vi "Accept.vi"(8 "Error in (no error)":errorcluster, 10 "Log in":T1 {"Priority" items=["EMERGENCY", "ALERT", "CRITICAL", "ERROR", "WARNING", "NOTICE", "INFO", "DEBUG"]}, 11 "LogFilterMessage in":refnum<class "LogFilterMessage.lvclass">) -> (0 "Error out":errorcluster, 2 "Accept":bool, 3 "LogFilterMessage out":refnum<class "LogFilterMessage.lvclass">)   [LabVIEW 2011, in "LogFilterMessage.lvclass"]
uses:
  LogFilterMessage.lvclass
  Log/LogCluster.ctl
  Log/PrioritiesRing.ctl
  LogFilterMessage.lvclass/LogFilterMessage.ctl
  <vilib>/regexp/Match Regular Expression.xnode
  Log/Log.lvclass
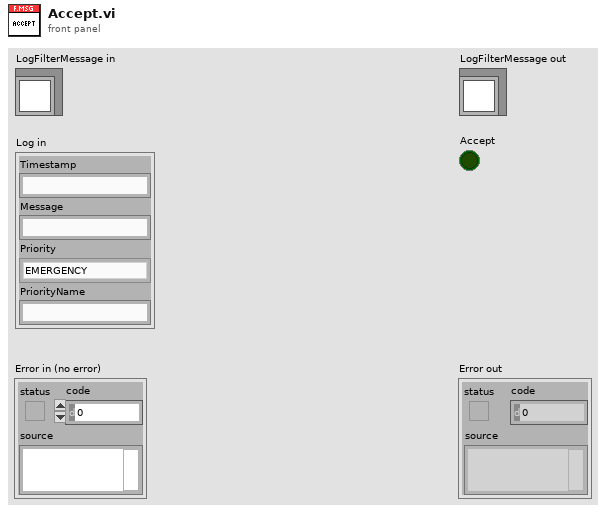
[diagram p1: front panel]
types:
  T1 = typedef "Log.lvclass/LogCluster.ctl" = cluster{"Timestamp":string, "Message":string, "Priority":T2, "PriorityName":string}
  T2 = typedef "Log.lvclass/PrioritiesRing.ctl" = u32
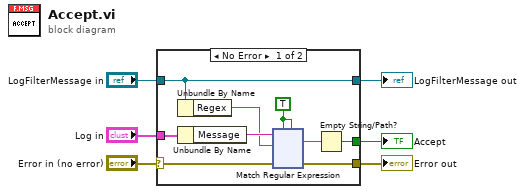
[diagram p0: block diagram]
diagram:
  n1 = case shown="No Error" "Error in (no error)" {
    selector: "Error in (no error)" -> [w11 w128]
    tunnel: [w10 w128] -> w5
    tunnel: [w13 w127] -> w3
    tunnel: "LogFilterMessage in" -> [w13 w127]
    tunnel: "Log in" -> [w15 _]
    tunnel: [w7 _] -> w1
    frame No Error {
      w9 = TRUE ("ignore case? (F)")
      n2 = Unbundle By Name(w13) -> ("Regex"=w12:string)
      n3 = Unbundle By Name(w15) -> ("Message"=w14:string)
      n4 = xnode "Match Regular Expression"("input string"=w14, "regular expression"=w12, "error in"=w11, "ignore case? (F)"=w9, "multiline? (F)"=w9) -> ("whole match"=w8:string, "error out"=w10:errorcluster)  [unwired: 1 in, 3 out]
      n5 = Empty String/Path?(string/path=w8) -> (empty?=w7:bool)
    }
    frame Error {
    }
  }
  "Error out" <- w5
  "LogFilterMessage out" <- w3
  "Accept" <- w1
